vi "Pre Launch Init.vi"(11 "MQTT-Client in":refnum<class "MQTT-Client.lvclass">) -> (0 "error out":errorcluster, 3 "MQTT-Client out":refnum<class "MQTT-Client.lvclass">)   [LabVIEW 2023, in "MQTT-Client.lvlib" / "MQTT-Client.lvclass"]
doc: "(<B>Filename</B>: Actor Framework.lvlib:Actor.lvclass:Pre Launch Init.vi)\n\nDefines behavior that occurs after the Launch Nested Actor method is invoked but before the actor's Actor Core method begins running.\n\nBy default, this method does nothing. A descendant class may override it to define behavior."
uses:
  MQTT-Client.lvclass
  MQTT-Client.lvclass/MQTT-Client.ctl
  <vilib>/ActorFramework/Actor/Actor.lvclass
  Config.ctl
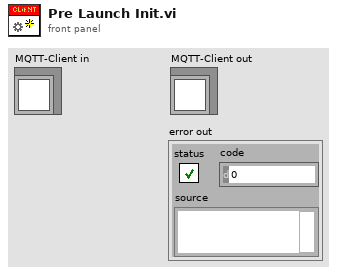
[diagram p1: front panel]
types:
  T1 = typedef "MQTT-Client.lvlib/MQTT-Client.lvclass/Config.ctl" = cluster{"scheduling":i32, "payload":string}
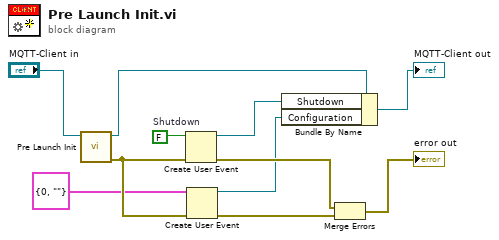
[diagram p0: block diagram]
diagram:
  w10 = FALSE  # Shutdown
  n1 = call-parent "Pre Launch Init.vi"("Actor in"="MQTT-Client in") -> ("error out"=w6:errorcluster, "Actor out"=w8:refnum<class "MQTT-Client.lvclass">)  [unwired: 9 in]
  n2 = Create User Event(user event datatype=w10, error in=w6) -> (user event=w9:refnum<user-event>, error out=w3:errorcluster)
  n3 = Create User Event(user event datatype=T1 {"scheduling"=0, "payload"=""} ("Configuration"), error in=w6) -> (user event=w1:refnum<user-event>, error out=w4:errorcluster)
  n4 = Bundle By Name(cluster=w8, "Shutdown"=w9, "Configuration"=w1) -> (→"MQTT-Client out":refnum<class "MQTT-Client.lvclass">)
  n5 = Merge Errors(w3, w4) -> (→"error out":errorcluster)
